vi "Artiq Client Submit.vi"(0 "Kasli Wrapper in":refnum<class "Kasli Wrapper 2.0.lvclass">=refnum, 1 "Overwrite?":bool=TRUE, 11 "error in (no error)":errorcluster) -> (4 "Kasli Wrapper out":refnum<class "Kasli Wrapper 2.0.lvclass">, 6 "standard output":string, 8 "standard error":string, 10 "return code":i32, 15 "error out":errorcluster)   [LabVIEW 2020, in "CIRCUS_uServices.lvlib" / "Kasli Wrapper 2.0.lvlib" / "Kasli Wrapper 2.0.lvclass"]
doc: "This VI is used to submit (i.e. enqueue) a new ARTIQ script into the pipeline of the Master.\nIf the Dummy flag is set to True, the script is submitted with the artiq_run command, ignoring the connection with a master.\nDAQ flag is used for specifying if the connection with the DAQ should be established by the script or is done outside."
uses:
  Kasli Wrapper 2.0.lvclass
  TALOS/TALOS_PPL.lvlibp
  C:/Users/marco/Documents/GitHub_Lab/CIRCUS/TALOS/TALOS_PPL.lvlibp/Father of all uServices/Father of all uServices/Father of all uServices.lvclass
  C:/Users/marco/Documents/GitHub_Lab/CIRCUS/TALOS/TALOS_PPL.lvlibp/Ancestor/Ancestor/Ancestor.lvclass
  C:/Users/marco/Documents/GitHub_Lab/CIRCUS/TALOS/Actor Framework.lvlibp/1abvi3w/vi.lib/ActorFramework/Actor/Actor.lvclass
  C:/Users/marco/Documents/GitHub_Lab/CIRCUS/CIRCUS uServices et al/Kasli Wrapper 2.0/Kasli Wrapper 2.0.lvclass
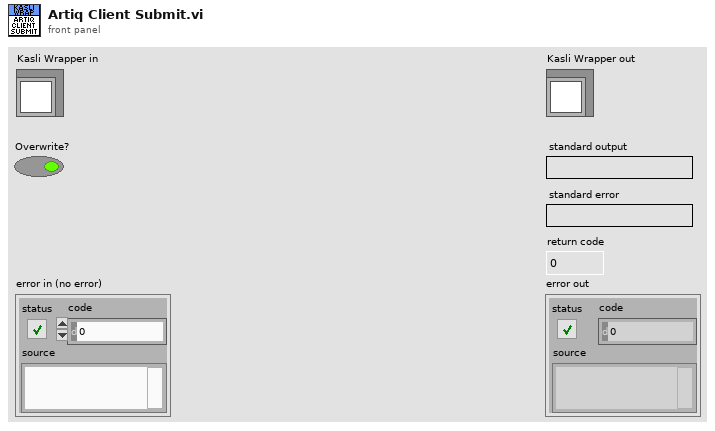
[diagram p1: front panel]
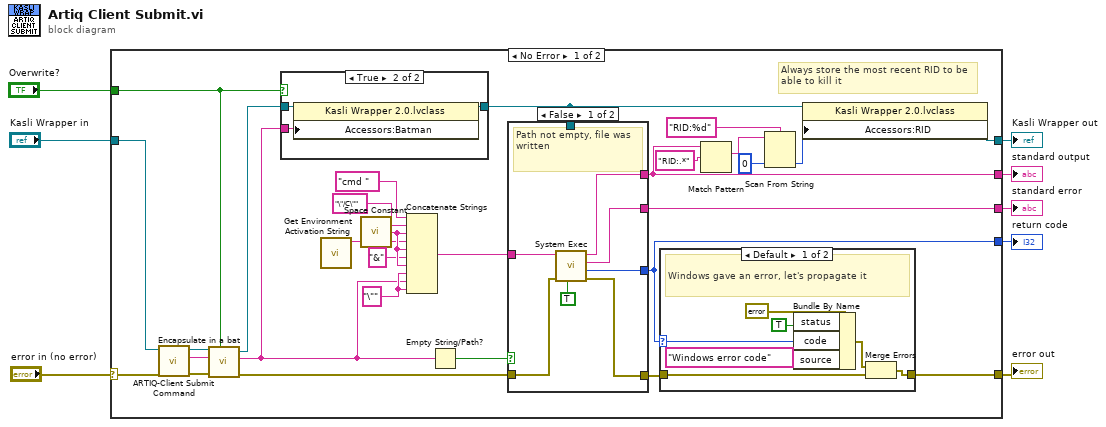
[diagram p0: block diagram]
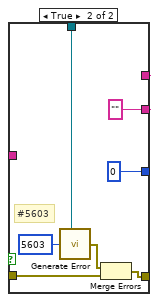
[diagram p4: hidden frame]
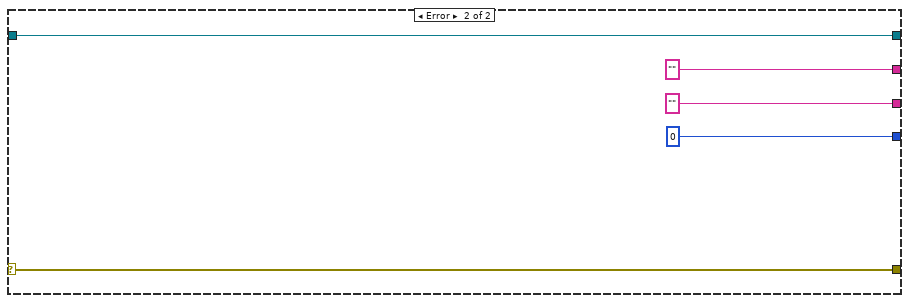
[diagram p5: hidden frame]
diagram:
  n1 = case shown="No Error" "error in (no error)" {
    selector: "error in (no error)" -> [w20 w68]
    tunnel: [w32 w68] -> w7
    tunnel: "Kasli Wrapper in" -> [w16 w67]
    tunnel: [w13 w67] -> w5
    tunnel: [w11 "" ("standard output")] -> w2
    tunnel: [w37 "" ("standard error")] -> w3
    tunnel: [w23 0 ("return code")] -> w4
    tunnel: "Overwrite?" -> [w15 _]
    frame No Error {
      w30 = "\"" ("string")
      # "Always store the most recent RID to be able to kill it"
      n2 = call-dynamic "ARTIQ-Client Submit Command.vi"("error in (no error)"=w20, "Kasli Wrapper 2.0 in"=w16) -> ("error out"=w19:errorcluster, "artiq-client submit"=w18:string, "Kasli Wrapper 2.0 out"=w17:refnum<class "Kasli Wrapper 2.0.lvclass">)  [unwired: 7 in]
      n3 = call-dynamic "Encapsulate in a bat.vi"("Overwrite?"=w15, "error in (no error)"=w19, "command"=w18, "Kasli Wrapper in"=w17) -> ("error out"=w36:errorcluster, "bat out"=w21:string, "Kasli Wrapper out"=w22:refnum<class "Kasli Wrapper 2.0.lvclass">)  [unwired: 5 in]
      n4 = case shown="True" w15 {
        tunnel: w22 -> [w38 w41]
        tunnel: [w38 w40] -> w14
        tunnel: w21 -> [_ w39]
        frame False {
        }
        frame True {
          n5 = property class="Kasli Wrapper 2.0.lvclass"(reference=w41, "Accessors:Batman"=w39) -> (reference out=w40:refnum<class "Kasli Wrapper 2.0.lvclass">)  [unwired: 1 in, 1 out]
        }
      }
      n6 = call "Get Environment Activation String.vi"() -> ("Conda Activation String"=w26:string)  [unwired: 10 in, 1 out]
      n7 = call <vilib>:"Space Constant.vi"() -> ("String"=w31:string)
      n8 = Concatenate Strings("cmd " ("command line"), "\"/C\"", w31, w26, w31, "&" ("string"), w31, w30, w21, w30) -> (w34:string)
      n9 = Empty String/Path?(string/path=w21) -> (empty?=w35:bool)
      n10 = case shown="False" w35 {
        tunnel: w34 -> [w55 _]
        tunnel: [w54 w57] -> w33
        tunnel: [w53 w63] -> w11
        tunnel: [w52 w63] -> w37
        tunnel: [w51 0 ("return code")] -> w23
        tunnel: w36 -> [w50 w59]
        tunnel: w14 -> [_ w61]
        frame False {
          # "Path not empty, file was written"
          n11 = call <vilib>:"System Exec.vi"("run minimized? (F)"=TRUE, "error in (no error)"=w50, "command line"=w55) -> ("error out"=w54:errorcluster, "return code"=w51:i32, "standard error"=w52:string, "standard output"=w53:string)  [unwired: 5 in]
        }
        frame True {
          w63 = "" ("standard output")
          # "#5603"
          n12 = call "Generate Error.vi"("Class"=w61, "Error Code"=5603) -> ("error out"=w58:errorcluster)  [unwired: 5 in]
          n13 = Merge Errors(w58, w59) -> (w57:errorcluster)
        }
      }
      n14 = case shown="Default" w23 {
        selector: w23 -> [w47 _]
        tunnel: w33 -> [w44 w49]
        tunnel: [w43 w49] -> w32
        frame Default {
          # "Windows gave an error, let's propagate it"
          n15 = Bundle By Name(cluster=errorcluster {"status"=FALSE, "code"=0, "source"=""} ("error constant"), "status"=TRUE, "code"=w47, "source"="Windows error code") -> (w45:errorcluster)
          n16 = Merge Errors(w45, w44) -> (w43:errorcluster)
        }
        frame 0 {
          # "Error code is OK"
        }
      }
      n17 = Match Pattern(string=w11, regular expression="RID:.*") -> (match substring=w10:string)  [unwired: 1 in, 3 out]
      n18 = Scan From String(format string="RID:%d", input string=w10, default 1=u32 0 ("RID")) -> (output 1=w12:u32)  [unwired: 2 in, 3 out]
      n19 = property class="Kasli Wrapper 2.0.lvclass"(reference=w14, "Accessors:RID"=w12) -> (reference out=w13:refnum<class "Kasli Wrapper 2.0.lvclass">)  [unwired: 1 in, 1 out]
    }
    frame Error {
    }
  }
  "Kasli Wrapper out" <- w5
  "error out" <- w7
  "return code" <- w4
  "standard error" <- w3
  "standard output" <- w2
